vi "Analog Write.vi"   [LabVIEW 2020, in "LMH-LINX.lvlib"]
uses:
  LMH-LINX.lvlib
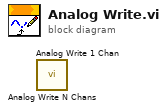
[diagram p0: block diagram]
diagram:
  n1 = call "Analog Write N Chans.vi"() -> ()  [unwired: 10 in, 2 out]
  n2 = call "Analog Write 1 Chan.vi"() -> ()  [unwired: 10 in, 2 out]
